vi "4_3.vi"() -> ()   [LabVIEW 2012]
panel:
  in  "stop":bool
  in  "OK Button":bool
  out "Numeric 2":dbl
  in  "Numeric":dbl
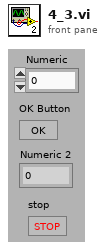
[diagram p1: front panel]
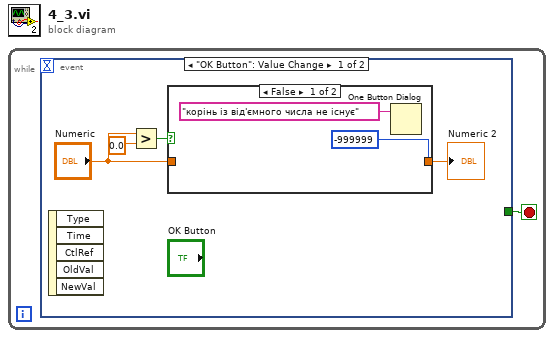
[diagram p0: block diagram]
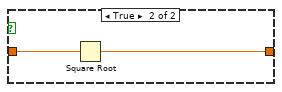
[diagram p2: hidden frame]
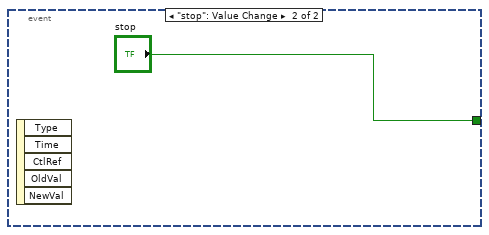
[diagram p3: hidden frame]
diagram:
  n1 = while {
    stop <- w1 stop-if-true
    n2 = event shown="[0] \"OK Button\": Value Change" {
      selector: _ -> [_ _]
      dyn-events: _ -> [_ _]
      timeout: _ -> [_ _]
      tunnel: [_ "stop"] -> w1
      event "OK Button": Value Change {
        n3 = event-data() -> ()  [unwired: 1 in, 5 out]
        n4 = Greater?(x="Numeric", y=0.0) -> (0:w4:bool)
        n5 = case shown="False" w4 {
          tunnel: "Numeric" -> [_ w9]
          tunnel: [-999999 w8] -> w2
          frame False {
            n6 = One Button Dialog(message="корінь із від'ємного числа не існує") -> ()  [unwired: 1 in, 1 out]
          }
          frame True {
            n7 = Square Root(x=w9) -> (sqrt(x)=w8:dbl)
          }
        }
        "Numeric 2" <- w2
      }
      event "stop": Value Change {
        n8 = event-data() -> ()  [unwired: 1 in, 5 out]
      }
    }
  }
